vi "EventsRobotsStuck.vi"(7 "FPS":dbl, 8 "Time":enum16{"Azul", "Amarelo"}(ring) caption="Enum", 9 "Detection Frame":T1 {"robots_blue"."height" format="%+4.3f"; "robots_blue"."pixel_y" format="%+4.3f"; "robots_blue"."pixel_x" format="%+4.3f"; "robots_blue"."orientation" format="%+4.3f"; "robots_blue"."y" format="%+4.3f"; "robots_blue"."confidence" format="%4.3f"; "robots_blue"."x" format="%+4.3f"; "robots_yellow"."height" format="%+4.3f"; "robots_yellow"."pixel_y" format="%+4.3f"; "robots_yellow"."pixel_x" format="%+4.3f"; "robots_yellow"."orientation" format="%+4.3f"; "robots_yellow"."y" format="%+4.3f"; "robots_yellow"."confidence" format="%4.3f"; "robots_yellow"."x" format="%+4.3f"}, 11 "IA State Input":T5) -> (2 "Robots stuck":cluster{"id":u32, dbl}[](array[cluster]), 3 "Is there any robot stuck?":bool)   [LabVIEW 2017]
uses:
  Core/AI Input.ctl
  Core/AI Robot.ctl
  Intel/Functions Enum.ctl
  Intel/AttackerStates.ctl
  Path Planning/RRT/PathDests.ctl
  Path Planning/RRT/PathDest.ctl
  Core/AI Ball.ctl
  Core/Field Size.ctl
  Core/AI Judge.ctl
  Intel/Command Enum.ctl
  Events.ctl
  SSL Detection Frame.ctl
  SSL Detection Robot.ctl
  <vilib>/Analysis/Matrix/Datatypes/RealMatrix.ctl
  SSL Detection Ball.ctl
  <vilib>/Analysis/Matrix/NI_Matrix.lvlib
panel:
  out "empty?":bool
  out "Boolean":bool=TRUE
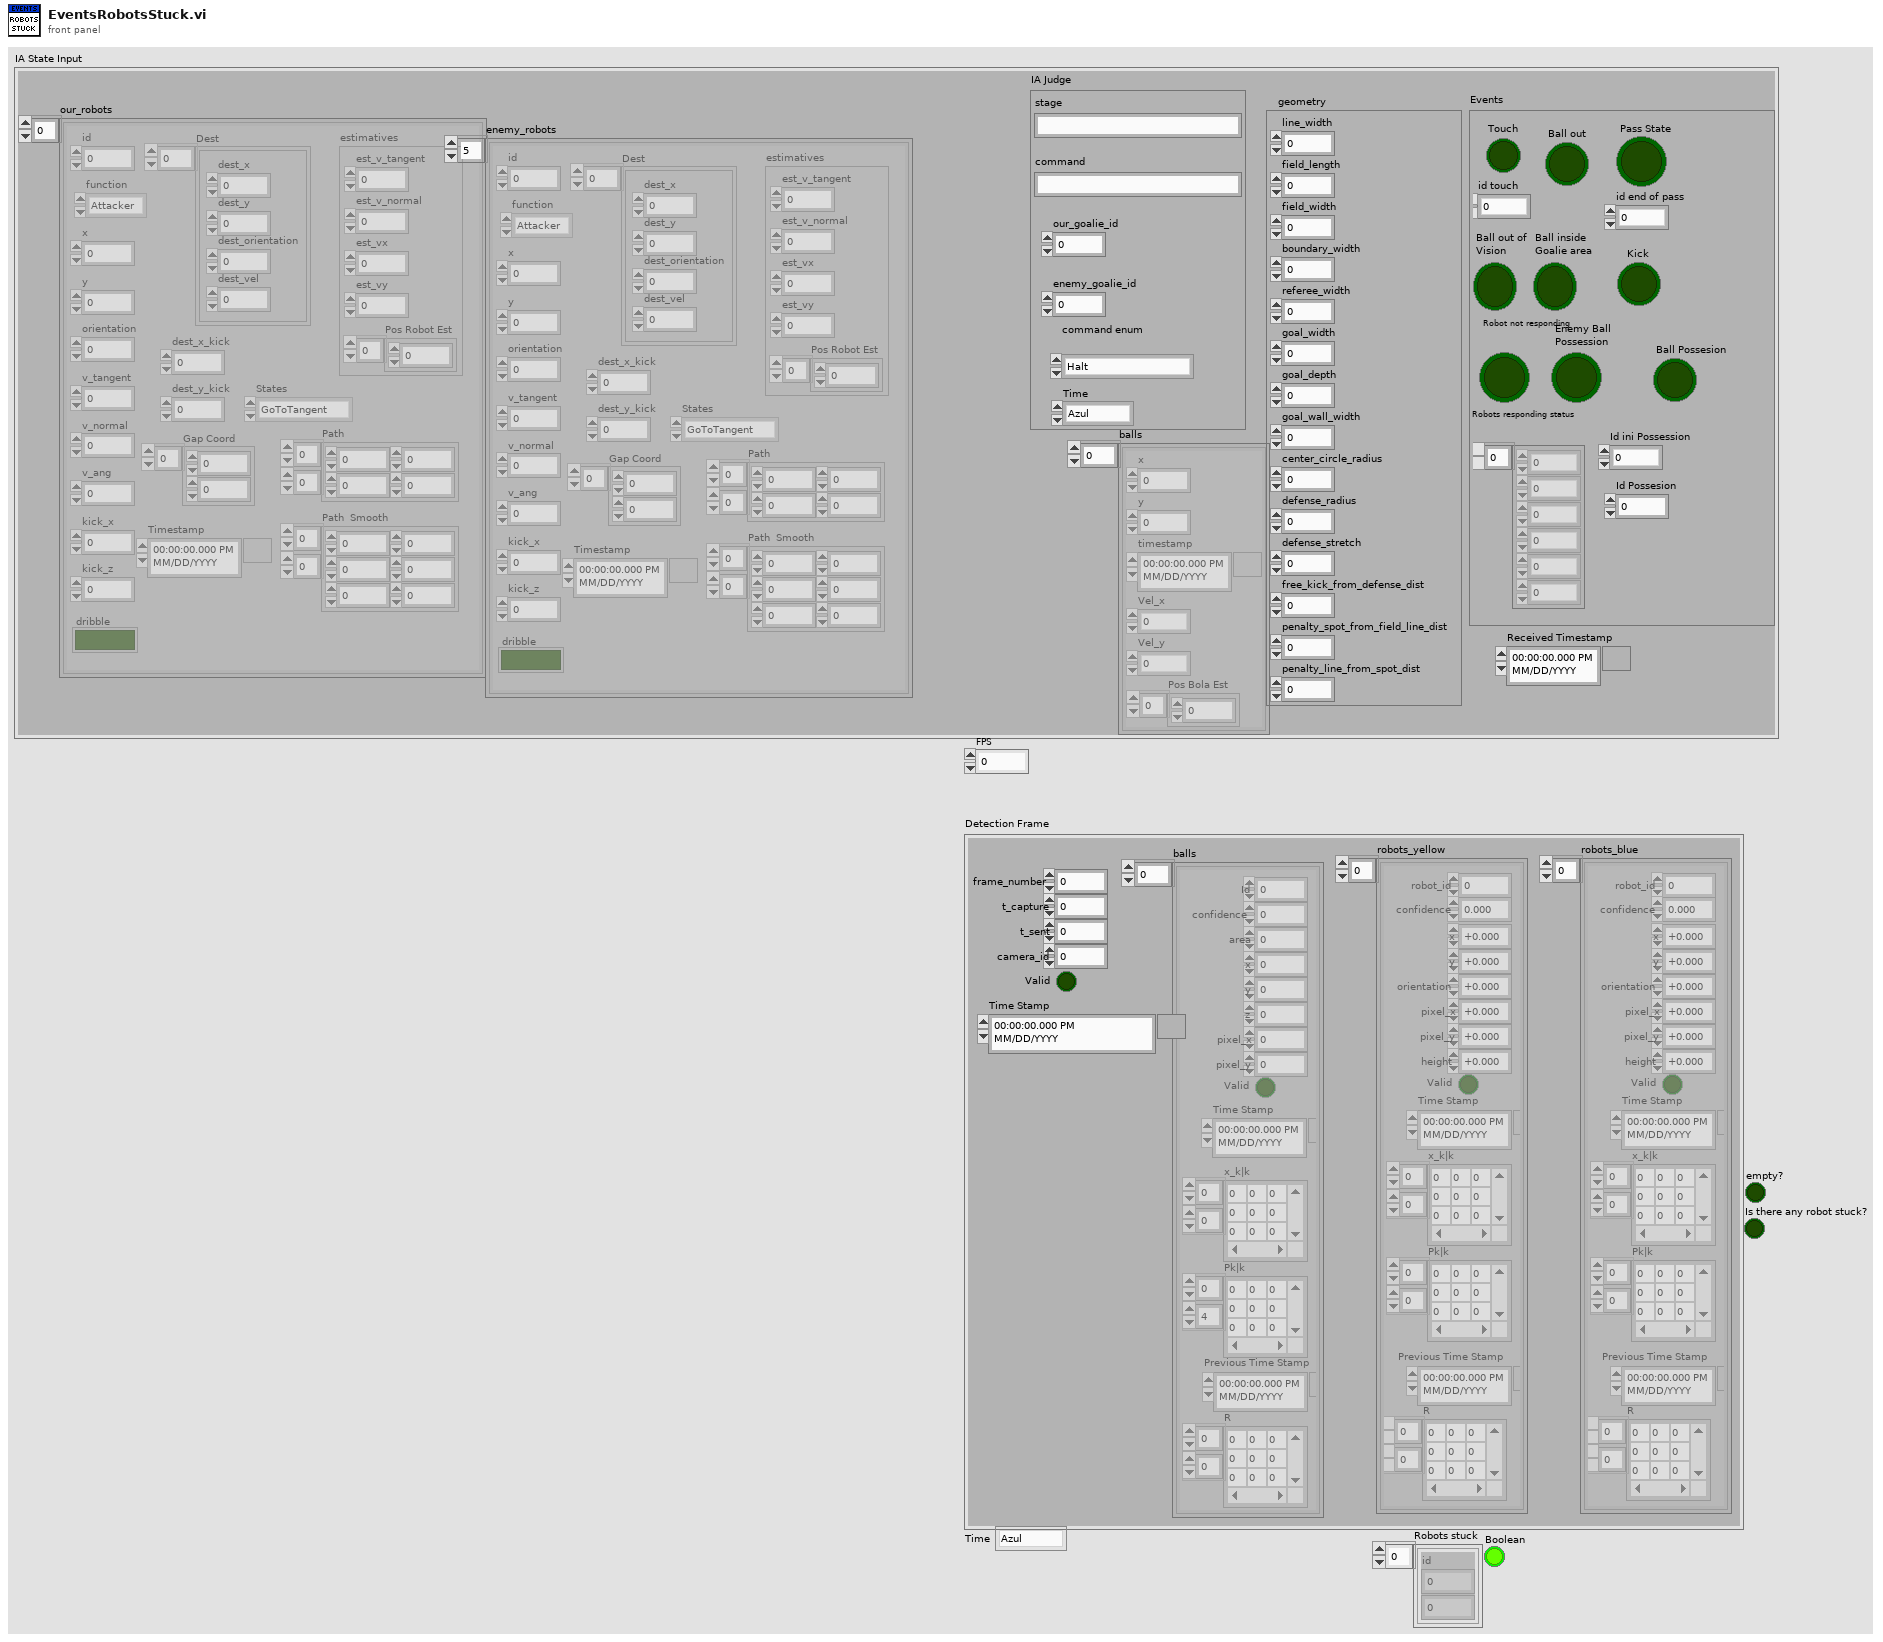
[diagram p1: front panel]
types:
  T1 = typedef "SSL Detection Frame.ctl" = cluster{"frame_number":u32, "t_capture":dbl, "t_sent":dbl, "camera_id":u32, "robots_yellow":T2[], "robots_blue":T2[], "balls":T4[], "Valid":bool, "Time Stamp":timestamp}
  T2 = typedef "SSL Detection Robot.ctl" = cluster{"x":sgl, "robot_id":u32, "confidence":sgl, "y":sgl, "orientation":sgl, "pixel_x":sgl, "pixel_y":sgl, "height":sgl, "Valid":bool, "Time Stamp":timestamp, "x_k|k":T3, "Pk|k":T3, "Previous Time Stamp":timestamp, "R":T3}
  T3 = typedef "NI_Matrix.lvlib/RealMatrix.ctl" = dbl[][]
  T4 = typedef "SSL Detection Ball.ctl" = cluster{"x":sgl, "area":u32, "confidence":sgl, "y":sgl, "z":sgl, "pixel_x":sgl, "pixel_y":sgl, "Valid":bool, "Time Stamp":timestamp, "x_k|k":T3, "Pk|k":T3, "Id":u32, "Previous Time Stamp":timestamp, "R":T3}
  T5 = typedef "AI Input.ctl" = cluster{"our_robots":T6[], "enemy_robots":T6[], "balls":T11[], "geometry":T12, "IA Judge":T13, "Received Timestamp":timestamp, "Events":T15}
  T6 = typedef "AI Robot.ctl" = cluster{"id":u32, "function":T7, "x":dbl, "y":dbl, "orientation":dbl, "v_tangent":dbl, "v_normal":dbl, "v_ang":dbl, "kick_x":dbl, "kick_z":dbl, "dribble":bool, "Timestamp":timestamp, "estimatives":cluster{"est_v_tangent":dbl, "est_v_normal":dbl, "est_vx":dbl, "est_vy":dbl, "Pos Robot Est":dbl[]}, "dest_x_kick":dbl, "dest_y_kick":dbl, "Gap Coord":dbl[], "States":T8, "Path ":dbl[][], "Path  Smooth":dbl[][], "Dest":T9}
  T7 = typedef "Functions Enum.ctl" = enum16{"Attacker", "Goalie", "Defender", "Striker", "Goto 0", "Dummy", "Kicker", "ZigZag"}
  T8 = typedef "AttackerStates.ctl" = enum16{"Pass", "GoToTangent", "BallGetting", "GoToKick", ""}
  T9 = typedef "PathDests.ctl" = T10[]
  T10 = typedef "PathDest.ctl" = cluster{"dest_x":dbl, "dest_y":dbl, "dest_orientation":dbl, "dest_vel":dbl}
  T11 = typedef "AI Ball.ctl" = cluster{"x":dbl, "y":dbl, "timestamp":timestamp, "Vel_x":dbl, "Vel_y":dbl, "Pos Bola Est":dbl[]}
  T12 = typedef "Field Size.ctl" = cluster{"line_width":u32, "field_length":u32, "field_width":u32, "boundary_width":u32, "referee_width":u32, "goal_width":u32, "goal_depth":u32, "goal_wall_width":u32, "center_circle_radius":u32, "defense_radius":u32, "defense_stretch":u32, "free_kick_from_defense_dist":u32, "penalty_spot_from_field_line_dist":u32, "penalty_line_from_spot_dist":u32}
  T13 = typedef "AI Judge.ctl" = cluster{"stage":string, "command":string, "our_goalie_id":dbl, "enemy_goalie_id":dbl, "command enum":T14, "Time":enum16{"Azul", "Amarelo"}}
  T14 = typedef "Command Enum.ctl" = enum16{"Halt", "Stop", "Force Start", "PKA Normal Start", "Prepare Kickoff Ally", "PKE Normal Start", "Prepare Kickoff Enemy", "Prepare Penalty Ally", "PPA Normal Start", "Prepare Penalty Enemy", "PPE Normal Start", "Direct Free Enemy", "Direct Free Ally", "Indirect Free Enemy", "Indirect Free Ally", "Timeout Enemy", "Timeout Ally", "Goal Enemy", "Goal Ally", "Ball Placement Enemy", "Ball Placement Ally", "Normal Half Time", "Extra Time Break", "Extra Half Time", "None", "Post Game"}
  T15 = typedef "Events.ctl" = cluster{"Touch":bool, "Ball out":bool, "id touch":dbl, "Ball out of \nVision":bool, "Ball inside \nGoalie area":bool, "Robot not responding":bool, "Robots responding status":dbl[], "Enemy Ball \nPossession":bool, "Pass State":bool, "id end of pass":dbl, "Kick":bool, "Id ini Possession":dbl, "Ball Possesion":bool, "Id Possesion":dbl}
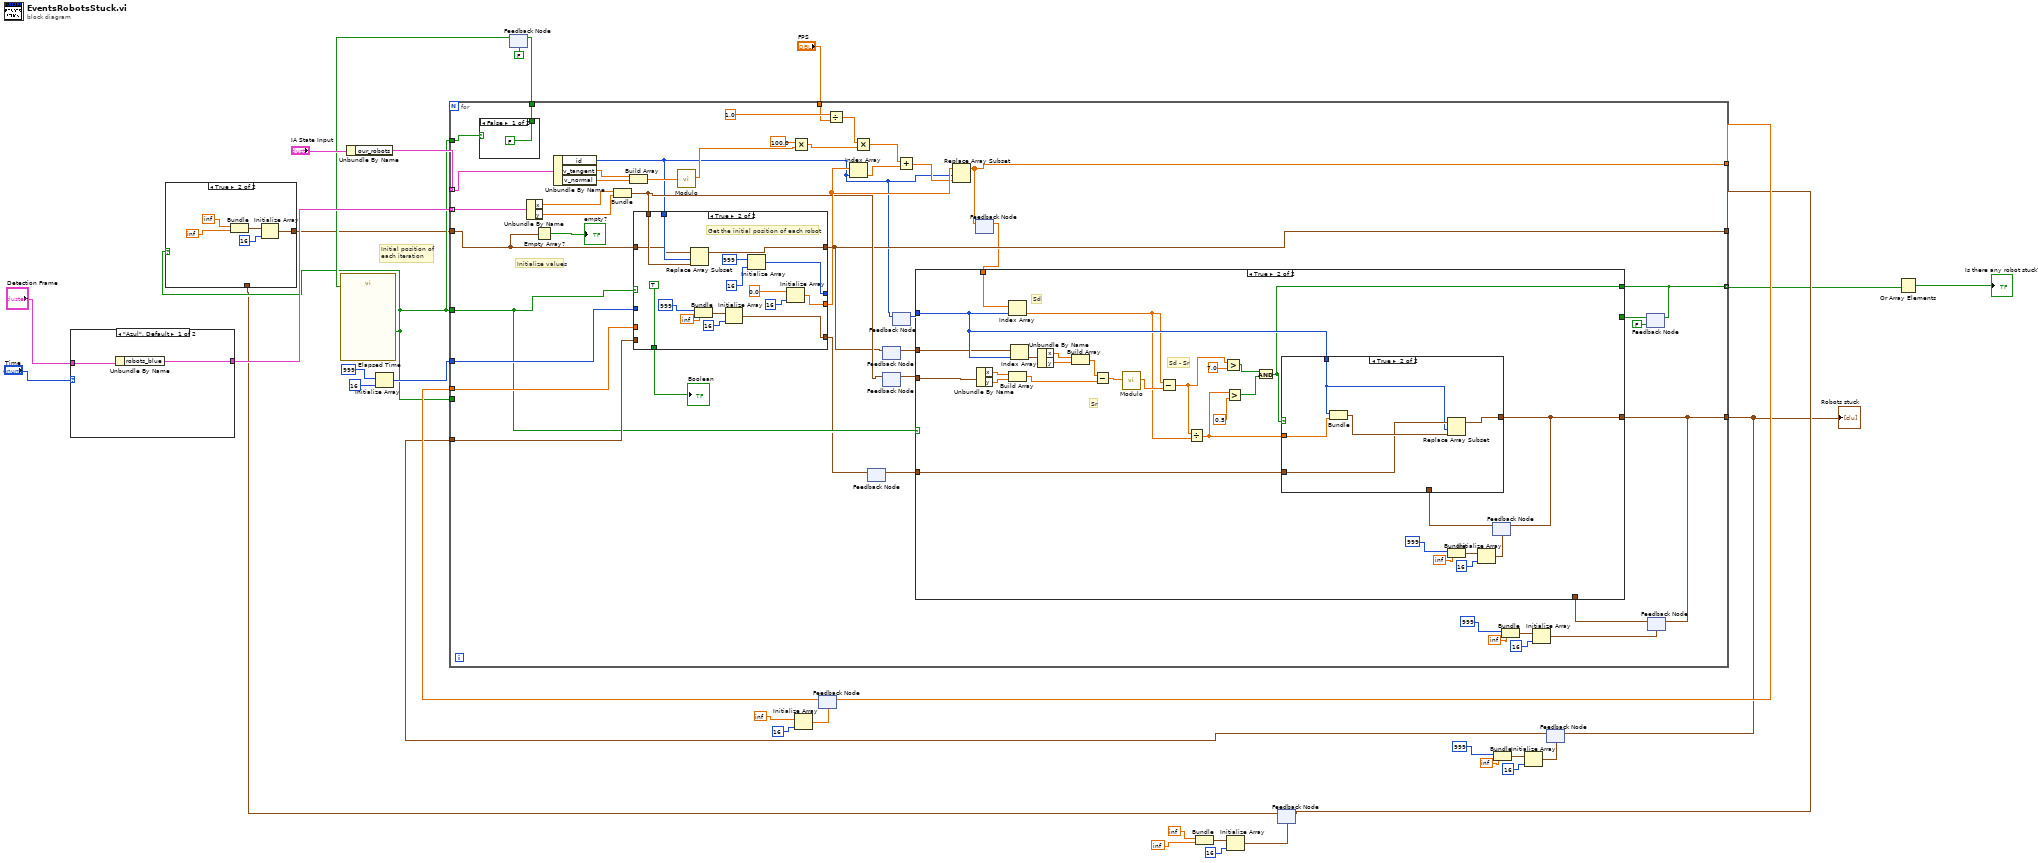
[diagram p0: block diagram]
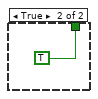
[diagram p5: hidden frame]
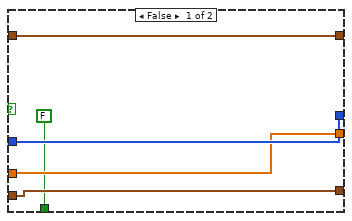
[diagram p6: hidden frame]
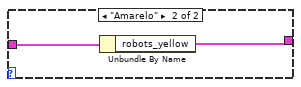
[diagram p7: hidden frame]
diagram:
  # "Initial position of\neach iteration"
  n1 = case shown="\"Azul\", Default" "Time" {
    tunnel: "Detection Frame" -> [w37 w39]
    tunnel: [w36 w38] -> w28
    frame "Azul", Default {
      n2 = Unbundle By Name(w37) -> ("robots_blue"=w36:T2[])
    }
    frame "Amarelo" {
      n3 = Unbundle By Name(w39) -> ("robots_yellow"=w38:T2[])
    }
  }
  n4 = Unbundle By Name("IA State Input") -> ("our_robots"=w34:T6[])
  n5 = Initialize Array(999 ("dimension size"), 16 ("dimension size")) -> (w25:i32[])
  n6 = feedback #1(FALSE) -> (w14:bool)
  n7 = call "Elapsed Time"("Reset"=w14) -> ("Time has Elapsed"=w6:bool)  [unwired: 11 in, 7 out]
  n8 = Initialize Array(inf ("y"), 16 ("dimension size")) -> (w17:dbl[])
  n9 = feedback #2(w17) -> (w31:dbl[])
  n10 = Bundle("x"=sgl inf, "y"=sgl inf) -> (w10:cluster{"x":sgl, "y":sgl})  [unwired: 1 in]
  n11 = Initialize Array(w10, 16 ("dimension size")) -> (w7:cluster{"x":sgl, "y":sgl}[])
  n12 = feedback #3(w7) -> (w4:cluster{"x":sgl, "y":sgl}[])
  n13 = case shown="True" w6 {
    tunnel: [w40 w41] -> w5
    tunnel: w4 -> [w40 _]
    frame False {
    }
    frame True {
      n14 = Bundle("x"=sgl inf, "y"=sgl inf) -> (w44:cluster{"x":sgl, "y":sgl})  [unwired: 1 in]
      n15 = Initialize Array(w44, 16 ("dimension size")) -> (w41:cluster{"x":sgl, "y":sgl}[])
    }
  }
  n16 = Bundle("dimension size"=999, "y"=inf) -> (w23:cluster{"dimension size":i32, "y":dbl})  [unwired: 1 in]
  n17 = Initialize Array(w23, 16 ("dimension size")) -> (w21:cluster{"dimension size":i32, "y":dbl}[])
  n18 = feedback #4(w21) -> (w13:cluster{"dimension size":i32, "y":dbl}[])
  n19 = for {
    tunnel: w34 -> [w80] mode=indexing
    tunnel: w31 -> [w91]
    tunnel: w25 -> [w70]
    tunnel: w6 -> [w66]
    tunnel: "FPS" -> [w85]
    tunnel: [w47] -> w32
    tunnel: w6 -> [_]
    tunnel: w13 -> [w79]
    tunnel: [w65] -> w3
    tunnel: w28 -> [w78] mode=indexing
    tunnel: w6 -> [w72]
    tunnel: [w71] -> w16
    tunnel: w5 -> [w68]
    tunnel: [w51] -> w12
    tunnel: [w63] -> w1 mode=indexing
    # "Initialize values"
    n20 = case shown="False" w72 {
      tunnel: [FALSE TRUE] -> w71
      frame False {
      }
      frame True {
      }
    }
    n21 = Unbundle By Name(w78) -> ("x"=w77:sgl, "y"=w76:sgl)
    n22 = Empty Array?(array=w68) -> (empty?=→"empty?":bool)
    n23 = Unbundle By Name(w80) -> ("id"=w49:u32, "v_tangent"=w90:dbl, "v_normal"=w89:dbl)
    n24 = Bundle("x"=w77, "y"=w76) -> (w53:cluster{"x":sgl, "y":sgl})  [unwired: 1 in]
    n25 = Build Array(w90, w89) -> (w88:dbl[])
    n26 = case shown="True" w66 {
      tunnel: w70 -> [w135 _]
      tunnel: w91 -> [w134 _]
      tunnel: [w135 w145] -> _
      tunnel: [w134 w143] -> w82
      tunnel: w53 -> [_ w149]
      tunnel: w49 -> [_ w151]
      tunnel: [w133 w150] -> w51
      tunnel: w68 -> [w133 w148]
      tunnel: w79 -> [w132 _]
      tunnel: [w132 w139] -> w55
      tunnel: [FALSE TRUE] -> w69
      frame False {
      }
      frame True {
        # "Get the initial position of each robot"
        n27 = Replace Array Subset(array=w148, new element=w149, index=w151) -> (w150:cluster{"x":sgl, "y":sgl}[])
        n28 = Bundle("ID"=999, "Relative error"=inf) -> (w141:cluster{"ID":i32, "Relative error":dbl})  [unwired: 1 in]
        n29 = Initialize Array(w141, 16 ("dimension size")) -> (w139:cluster{"ID":i32, "Relative error":dbl}[])
        n30 = Initialize Array(999 ("dimension size"), 16 ("dimension size")) -> (w145:i32[])
        n31 = Initialize Array(0.0 ("element"), 16 ("dimension size")) -> (w143:dbl[])
      }
    }
    "Boolean" <- w69
    n32 = call "Modulo.vi"("2D vector"=w88) -> ("Modulo"=w75:dbl)  [unwired: 10 in]
    n33 = Multiply(x=100.0, y=w75) -> (x*y=w73:dbl)
    n34 = Divide(x=1.0, y=w85) -> (x/y=w84:dbl)
    n35 = Index Array(array=w82, index=w49) -> (element=w87:dbl)
    n36 = Multiply(x=w84, y=w73) -> (x*y=w83:dbl)
    n37 = feedback #5() -> (w54:cluster{"ID":i32, "Relative error":dbl}[])  [unwired: 1 in]
    n38 = feedback-in #5(w55) -> ()
    n39 = feedback #6() -> (w50:cluster{"x":sgl, "y":sgl}[])  [unwired: 1 in]
    n40 = feedback-in #6(w51) -> ()
    n41 = feedback #7() -> (w52:cluster{"x":sgl, "y":sgl})  [unwired: 1 in]
    n42 = feedback-in #7(w53) -> ()
    n43 = feedback #8() -> (w48:u32)  [unwired: 1 in]
    n44 = feedback-in #8(w49) -> ()
    n45 = Add(x=w83, y=w87) -> (x+y=w81:dbl)
    n46 = Replace Array Subset(array=w82, new element=w81, index=w49) -> (w47:dbl[])
    n47 = feedback #9() -> (w46:dbl[])  [unwired: 1 in]
    n48 = feedback-in #9(w47) -> ()
    n49 = Bundle("dimension size"=999, "y"=inf) -> (w59:cluster{"dimension size":i32, "y":dbl})  [unwired: 1 in]
    n50 = Initialize Array(w59, 16 ("dimension size")) -> (w56:cluster{"dimension size":i32, "y":dbl}[])
    n51 = feedback #10(FALSE) -> (w62:bool)
    n52 = feedback #11(w56) -> (w64:cluster{"dimension size":i32, "y":dbl}[])
    n53 = case shown="True" w66 {
      tunnel: w46 -> [_ w122]
      tunnel: w48 -> [_ w121]
      tunnel: w50 -> [_ w120]
      tunnel: w54 -> [_ w119]
      tunnel: w52 -> [_ w118]
      tunnel: [w93 w117] -> w65
      tunnel: [w92 w116] -> w63
      tunnel: w64 -> [w93 _]
      tunnel: w62 -> [w92 _]
      frame False {
      }
      frame True {
        # "Sr"
        # "Sd"
        # "Sd - Sr"
        n54 = Unbundle By Name(w118) -> ("x"=w111:sgl, "y"=w110:sgl)
        n55 = Index Array(array=w122, index=w121) -> (element=w105:dbl)
        n56 = Build Array(w111, w110) -> (w108:sgl[])
        n57 = Index Array(array=w120, index=w121) -> (element=w115:cluster{"x":sgl, "y":sgl})
        n58 = Unbundle By Name(w115) -> ("x"=w114:sgl, "y"=w113:sgl)
        n59 = Build Array(w114, w113) -> (w109:sgl[])
        n60 = Subtract(x=w109, y=w108) -> (x-y=w107:sgl[])
        n61 = call "Modulo.vi"("2D vector"=w107) -> ("Modulo"=w106:dbl)  [unwired: 10 in]
        n62 = Subtract(x=w105, y=w106) -> (x-y=w94:dbl)
        n63 = Divide(x=w94, y=w105) -> (x/y=w99:dbl)
        n64 = Greater?(x=w94, y=7.0) -> (0:w96:bool)
        n65 = Greater?(x=w99, y=0.5) -> (0:w97:bool)
        n66 = And(x=w96, y=w97) -> (x .and. y?=w116:bool)
        n67 = Bundle("dimension size"=999, "y"=inf) -> (w103:cluster{"dimension size":i32, "y":dbl})  [unwired: 1 in]
        n68 = Initialize Array(w103, 16 ("dimension size")) -> (w101:cluster{"dimension size":i32, "y":dbl}[])
        n69 = feedback #12(w101) -> (w112:cluster{"dimension size":i32, "y":dbl}[])
        n70 = case shown="True" w116 {
          tunnel: w121 -> [_ w124]
          tunnel: w99 -> [_ w128]
          tunnel: [w123 w127] -> w117
          tunnel: w112 -> [w123 _]
          tunnel: w119 -> [_ w125]
          frame False {
          }
          frame True {
            n71 = Bundle("id"=w124, w128) -> (w126:cluster{"id":u32, dbl})  [unwired: 1 in]
            n72 = Replace Array Subset(array=w125, new element=w126, index=w124) -> (w127:cluster{"ID":i32, "Relative error":dbl}[])
          }
        }
        n73 = feedback-in #12(w117) -> ()
      }
    }
    n74 = feedback-in #10(w63) -> ()
    n75 = feedback-in #11(w65) -> ()
  }
  "Robots stuck" <- w3
  n76 = feedback-in #1(w16) -> ()
  n77 = feedback-in #2(w32) -> ()
  n78 = feedback-in #3(w12) -> ()
  n79 = feedback-in #4(w3) -> ()
  n80 = Or Array Elements(Boolean array=w1) -> (logical OR=→"Is there any robot stuck?":bool)
